vi "EjemploGuardarGrafica.vi"() -> ()   [LabVIEW 2015]
panel:
  out "XY Graph":cluster{dbl[], dbl[]}(graph)
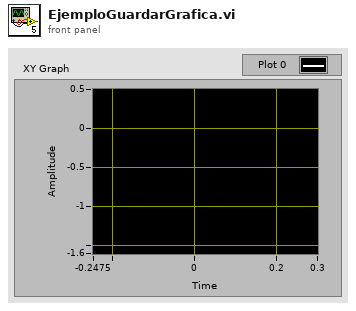
[diagram p1: front panel]
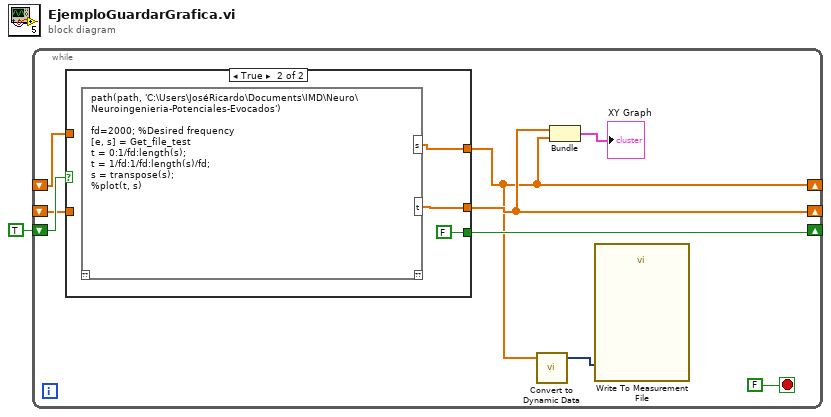
[diagram p0: block diagram]
diagram:
  n1 = while {
    shift-right: [w9] -> _
    shift-left: TRUE -> [w8]
    shift-right: [w2] -> _
    shift-left: _ -> [w7]
    shift-right: [w5] -> _
    shift-left: _ -> [w6]
    stop <- FALSE stop-if-true
    n2 = case shown="True" w8 {
      selector: w8 -> [w13 _]
      tunnel: [w12 w16] -> w2
      tunnel: [w13 FALSE] -> w9
      tunnel: w7 -> [w12 _]
      tunnel: [w11 w14] -> w5
      tunnel: w6 -> [w11 _]
      frame False {
      }
      frame True {
        n3 = script code="path(path, 'C:\\Users\\JoséRicardo\\Documents\\IMD\\Neuro\\Neuroingenieria-Potenciales-Evocados')\n\nfd=2000; %Desired frequency\n[e, s] = Get_file_test\nt = 0:1/fd:length(s);\nt = 1/fd:1/fd:length(s)/fd;\ns = transpose(s);\n%plot(t, s)"() -> ("s"=w16:dbl[], "t"=w14:dbl[])  [unwired: 1 in, 1 out]
      }
    }
    n4 = call "Convert to Dynamic Data"("Array"=w2) -> ("Dynamic Data Type"=w3:dynamicdata)  [unwired: 3 in]
    n5 = Bundle(w5, w2) -> (→"XY Graph":cluster{dbl[], dbl[]})  [unwired: 1 in]
    n6 = call "Write To Measurement File"("Signals"=w3) -> ()  [unwired: 16 in, 3 out]
  }
